vi "Pane MouseDown CB.vi"(4 "output cluster":T1, 5 "Event Data":T3, 6 "PaneRef":refnum<vi>, 7 "Event Common Data":cluster{"Source":T4, "Type":T5, "Time":u32} {"Source" items=["LabVIEW UI"=0, "ActiveX"=1, "User Event"=25]}) -> ()   [LabVIEW 2020]
uses:
  <vilib>/event_ctls.llb/eventsource.ctl
  <vilib>/event_ctls.llb/lveventtype.ctl
  <vilib>/Utility/miscctls.llb/LVPoint32TypeDef.ctl
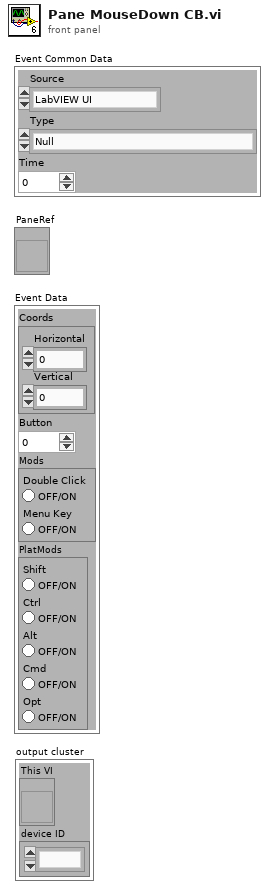
[diagram p1: front panel]
types:
  T1 = cluster{"This VI":refnum<vi>, "device ID":refnum<k1>}
  T2 = typedef "LVPoint32TypeDef.ctl" = cluster{"Horizontal":i32, "Vertical":i32}
  T3 = cluster{"Coords":T2, "Button":u16, "Mods":cluster{"Double Click":bool, "Menu Key":bool}, "PlatMods":cluster{"Shift":bool, "Ctrl":bool, "Alt":bool, "Cmd":bool, "Opt":bool}}
  T4 = typedef "eventsource.ctl" = u32
  T5 = typedef "lveventtype.ctl" = enum32{"Null", "Timeout", "Annotation Menu Selection", "Annotation Menu Selection?", "App Instance Close", "App Instance Close?", "Autoscale Range Change", "Bookmark Info Change", "Cell Edit", "Cell Edit?", "Cursor Grab", "Cursor Grab?", "Cursor Menu Selection", "Cursor Menu Selection?", "Cursor Move", "Cursor Release", "Data Change", "Direction Change", "Display State Change", "Drag Ended", "Drag Enter", "Drag Leave", "Drag Over", "Drag Source Update", "Drag Starting", "Drag Starting?", "Drop", "Exec State Change", "Key Down", "Key Down?", "Key Repeat", "Key Repeat?", "Key Up", "Listbox Double Click", "Menu Activation?", "Menu Selection (App)", "Menu Selection? (App)", "Menu Selection (User)", "Mouse Down", "Mouse Down?", "Mouse Enter", "Mouse Leave", "Mouse Move", "Mouse Up", "Mouse Wheel", "NI Security User Change (App)", "Pane Size", "Panel Close", "Panel Close?", "Panel Resize", "Plot Attribute Change", "Scale Range Change", "Shortcut Menu Activation?", "Shortcut Menu Selection (App)", "Shortcut Menu Selection? (App)", "Shortcut Menu Selection (User)", "Tree Double Click", "Tree Drag", "Tree Drag?", "Tree Drop", "Tree Drop?", "Tree Item Close", "Tree Item Close?", "Tree Item Open", "Tree Item Open?", "User Event", "Value Change"}
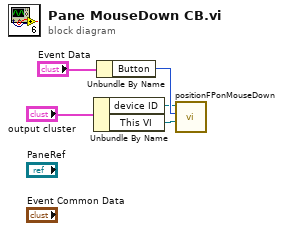
[diagram p0: block diagram]
diagram:
  n1 = Unbundle By Name("output cluster") -> ("device ID"=w1:refnum<k1>, "This VI"=w3:refnum<vi>)
  n2 = Unbundle By Name("Event Data") -> ("Button"=w2:u16)
  n3 = call "positionFPonMouseDown.vi"("VI Refnum"=w3, "Button (from Mouse Down event)"=w2, "mouse Device ID in"=w1) -> ()  [unwired: 7 in, 2 out]
